vi "AcquireImage.vi"(7 "Brightness":i64, 8 "Contrast":dbl, 9 "Image Src":T1, 10 "Session In":T2) -> (0 "error out":errorcluster, 2 "Image":T1(plugin-control), 3 "Session Out":T2)   [LabVIEW 2017]
uses:
  <vilib>/userdefined/High Color/IMAQdx.ctl
  <vilib>/vision/Image Controls.llb/IMAQ Image.ctl
  <vilib>/vision/driver/NI_Vision_Acquisition_Software.lvlib
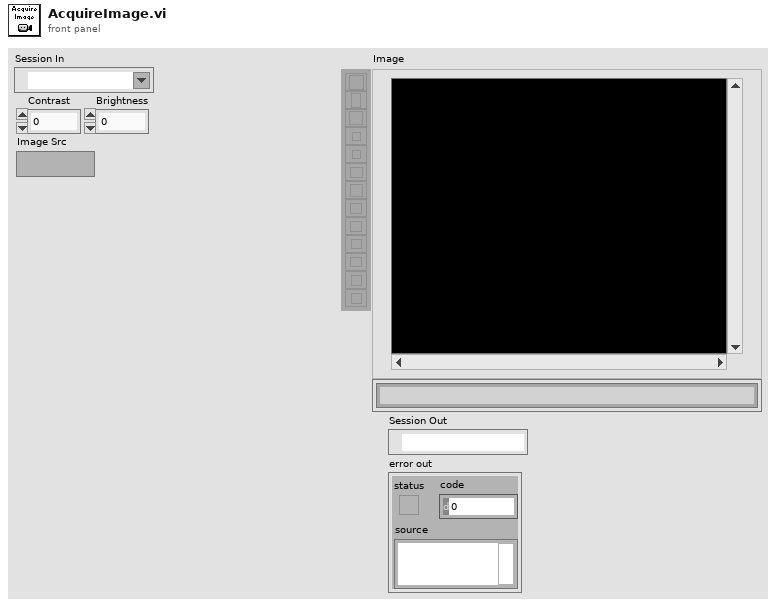
[diagram p1: front panel]
types:
  T1 = typedef "IMAQ Image.ctl" = refnum<image>
  T2 = typedef "IMAQdx.ctl" = refnum<k21>
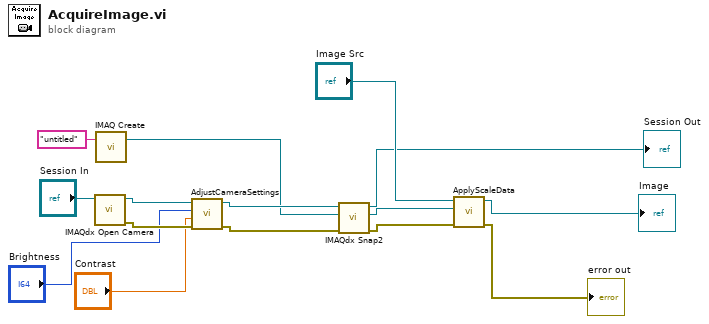
[diagram p0: block diagram]
diagram:
  n1 = call <vilib>:"IMAQdx Open Camera.vi"("Session In"="Session In") -> ("error out"=w10:errorcluster, "Session Out"=w13:T2)  [unwired: 9 in]
  n2 = call "IMAQ Create"("Image Name"="untitled") -> ("New Image"=w11:T1)  [unwired: 4 in, 1 out]
  n3 = call "AdjustCameraSettings.vi"("error in (no error)"=w10, "Contrast"="Contrast", "Brightness"="Brightness", "Session In"=w13) -> ("error out"=w9:errorcluster, "IMAQdx Session"=w12:T2)  [unwired: 4 in, 2 out]
  n4 = call <vilib>:"IMAQdx Snap2.vi"("error in"=w9, "Image In"=w11, "Session In"=w12) -> ("error out"=w4:errorcluster, "Image Out"=w5:T1, "Session Out"=→"Session Out":T2)  [unwired: 6 in]
  n5 = call "ApplyScaleData.vi"("error in (no error)"=w4, "Image Dst"=w5, "Image Src"="Image Src") -> ("error out"=→"error out":errorcluster, "Corrected Image"=→"Image":T1)  [unwired: 7 in]
